vi "Example Push Analog.vi"() -> ()   [LabVIEW 2015]
uses:
  Controls/SampleRateControlOut.ctl
  <vilib>/Utility/file.llb/Read Delimited Spreadsheet (DBL).vi
panel:
  in  "DAC Samplerate":T1
  in  "Calibrate":bool
  in  "Stop Button":bool
  in  "ADALM2000 URI:":string
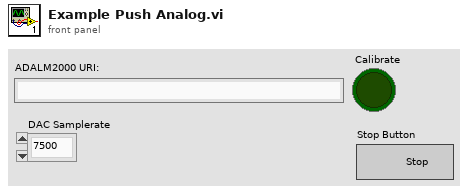
[diagram p1: front panel]
types:
  T1 = typedef "SampleRateControlOut.ctl" = enum16{"7500", "75000", "750000", "7500000", "75000000"}
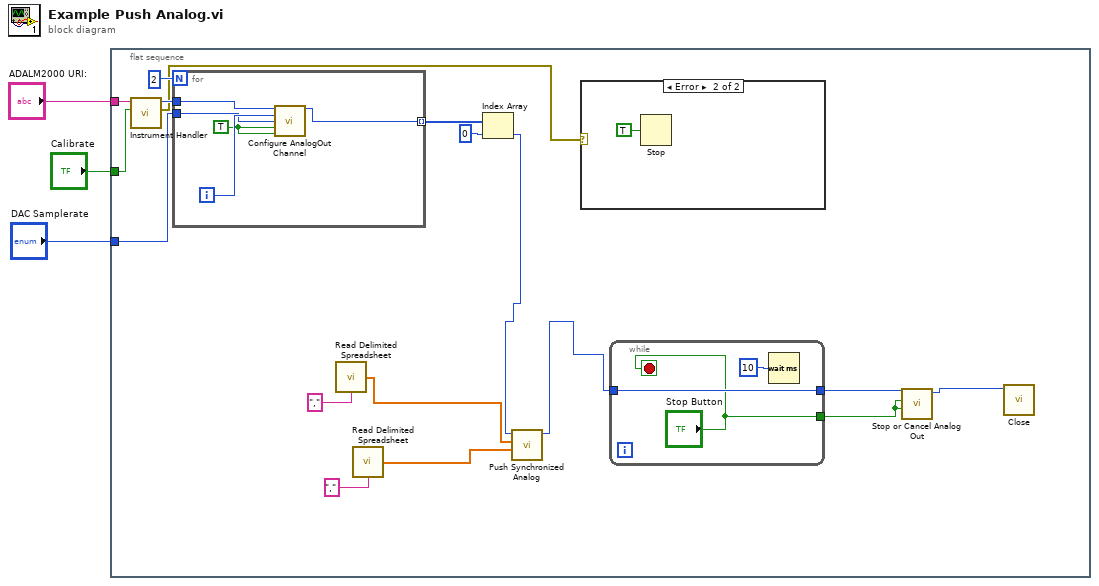
[diagram p0: block diagram]
diagram:
  n1 = flat-sequence {
    tunnel: "ADALM2000 URI:" -> [w17]
    tunnel: "Calibrate" -> [w16]
    tunnel: "DAC Samplerate" -> [w15]
    frame #0 {
      n2 = call "Instrument Handler.vi"("Calibrate"=w16, "ADALM2000 URI"=w17) -> ("error out"=w13:errorcluster, "ADALM2000 Handle"=w20:u32)  [unwired: 8 in]
      n3 = for {
        N: 2 -> [_]
        tunnel: w20 -> [w29]
        tunnel: [w25] -> w14 mode=indexing
        tunnel: w15 -> [w26]
        i -> [w28]
        w27 = TRUE ("Enable")
        n4 = call "Configure AnalogOut Channel.vi"("ADALM2000 Handler"=w29, "Channel"=w28, "Samplerate"=w26, "Enable"=w27, "Cyclic"=w27) -> ("ADALM2000 Handler 2"=w25:u32)  [unwired: 10 in]
      }
      n5 = call-poly <vilib>:"Read Delimited Spreadsheet.vi"("delimiter (\\t)"="," ("delimiter (\\t)")) -> ("first row"=w6:dbl[])  [unwired: 9 in, 5 out]
      n6 = call-poly <vilib>:"Read Delimited Spreadsheet.vi"("delimiter (\\t)"="," ("delimiter (\\t)")) -> ("first row"=w4:dbl[])  [unwired: 9 in, 5 out]
      n7 = Index Array(array=w14, index=0) -> (element=w7:u32)
      n8 = call "Push Synchronized Analog.vi"("samples chn 2"=w4, "samples chn 1"=w6, "ADALM2000 Handler"=w7) -> ("ADALM2000 Handler 2"=w8:u32)  [unwired: 8 in]
      n9 = case shown="Error" w13 {
        frame No Error {
        }
        frame Error {
          n10 = Stop(stop? (T)=TRUE) -> ()
        }
      }
      n11 = while {
        tunnel: w8 -> [w24]
        tunnel: [w24] -> w10
        tunnel: ["Stop Button"] -> w9
        stop <- "Stop Button" stop-if-true
        n12 = Wait (ms)(milliseconds to wait=u32 10) -> ()  [unwired: 1 out]
      }
      n13 = call "Stop or Cancel Analog Out.vi"("Stop"=w9, "Cancel"=w9, "ADALM2000 Handler"=w10) -> ("ADALM2000 Handler 2"=w11:u32)  [unwired: 8 in]
      n14 = call "Close.vi"("ADALM2000 Handler"=w11) -> ()  [unwired: 11 in]
    }
  }
